vi "groups_names_query_maker.vi"(2 "Small?":bool, 3 "Name Array":string[](array[string]), 4 "Group  Name":string) -> (0 "Parameters":string[](array[string]), 1 "Group and Names Query":string)   [LabVIEW 2013]
doc: "IMPORTANT: All input values can be left unwired, and the query will be modified to suit.\nTakes the experiment group and experiment names of a query and puts them in SQL syntax, in the following pattern:\n\"\n AND\n groups.group_names = '/Group Name/'\n AND\n (experiment_settings.tag = '/Name 1/'\n OR\n experiment_settings.tag = '/Name 2/')\""
uses:
  <userlib>/_OpenG.lib/string/string.llb/Trim Whitespace (String Array)__ogtk.vi
  <userlib>/_OpenG.lib/array/array.llb/Search 1D Array (String)__ogtk.vi
  <userlib>/_OpenG.lib/array/array.llb/Delete Elements from 1D Array (String)__ogtk.vi
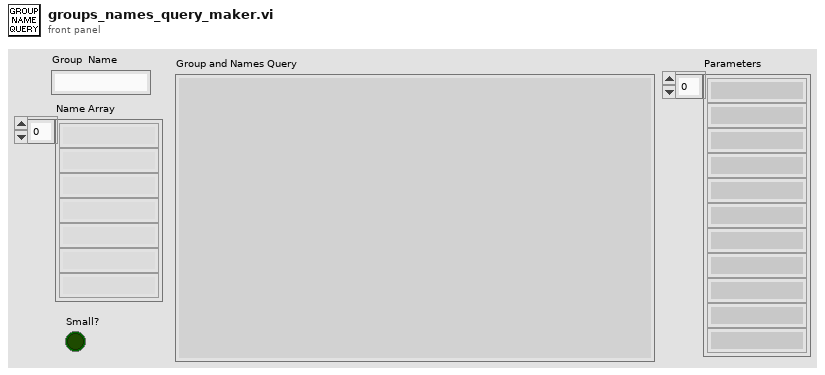
[diagram p1: front panel]
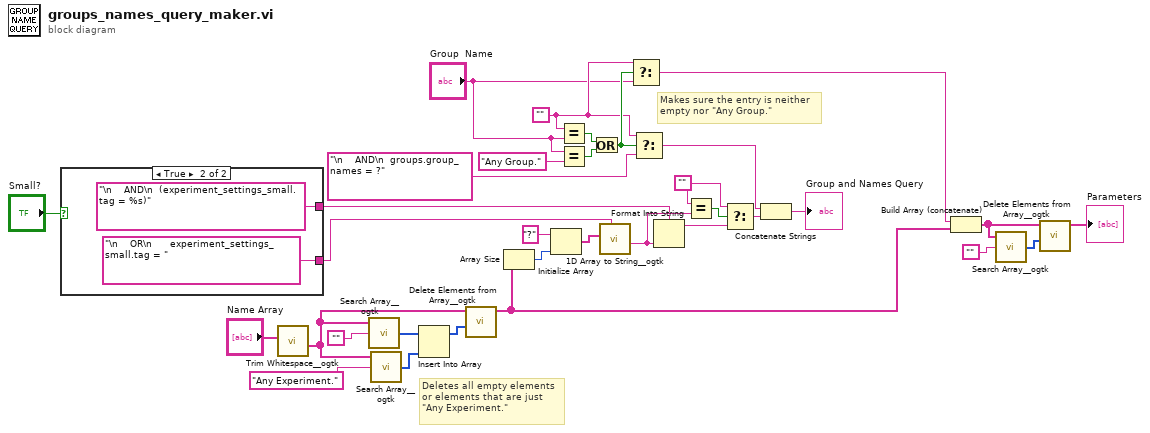
[diagram p0: block diagram]
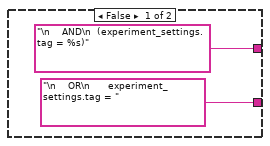
[diagram p2: hidden frame]
diagram:
  w12 = "" ("t")
  w29 = "" ("t")
  # "Makes sure the entry is neither\nempty nor \"Any Group.\""
  # "Deletes all empty elements\nor elements that are just\n\"Any Experiment.\""
  n1 = case shown="True" "Small?" {
    tunnel: ["\n    AND\n  (experiment_settings.tag = %s)" ("string") "\n    AND\n  (experiment_settings_small.tag = %s)" ("string")] -> w23
    tunnel: ["\n    OR\n      experiment_settings.tag = " ("string") "\n    OR\n      experiment_settings_small.tag = " ("string")] -> w22
    frame False {
    }
    frame True {
    }
  }
  n2 = call-poly <userlib>:"Trim Whitespace__ogtk.vi"("String in"="Name Array") -> ("String out"=w5:string[])  [unwired: 6 in]
  n3 = call-poly <userlib>:"Search Array__ogtk.vi"("Array"=w5, "Element Data"="") -> ("Indices of Elements"=w31:i32[])  [unwired: 7 in]
  n4 = call-poly <userlib>:"Search Array__ogtk.vi"("Array"=w5, "Element Data"="Any Experiment.") -> ("Indices of Elements"=w32:i32[])  [unwired: 7 in]
  n5 = Insert Into Array(array=w31, new element=w32) -> (w33:i32[])  [unwired: 1 in]
  n6 = call-poly <userlib>:"Delete Elements from Array__ogtk.vi"("indices"=w33, "array"=w5) -> ("array w/ subset deleted"=w8:string[])  [unwired: 8 in, 1 out]
  n7 = Array Size(array=w8) -> (size(s)=w9:i32)
  n8 = Initialize Array("?" ("Element Data"), w9) -> (w6:string[])
  n9 = Equal?(x=w12, y="Group  Name") -> (x = y?=w15:bool)
  n10 = Equal?(x="Group  Name", y="Any Group.") -> (x = y?=w16:bool)
  n11 = Or(x=w15, y=w16) -> (x .or. y?=w13:bool)
  n12 = call <userlib>:"1D Array to String__ogtk.vi"("delimiter (Tab)"=w22, "Array of Strings"=w6) -> ("delimited string"=w30:string)  [unwired: 9 in]
  n13 = Select(t=w12, s=w13, f="Group  Name") -> (s? t:f=w10:string)
  n14 = Select(t=w12, s=w13, f="\n    AND\n  groups.group_names = ?" ("string")) -> (s? t:f=w19:string)
  n15 = Format Into String(format string=w23, w30) -> (resulting string=w26:string)  [unwired: 2 in, 1 out]
  n16 = Equal?(x=w29, y=w30) -> (x = y?=w25:bool)
  n17 = Select(t=w29, s=w25, f=w26) -> (s? t:f=w20:string)
  n18 = Concatenate Strings(w19, w20) -> (→"Group and Names Query":string)
  n19 = Build Array (concatenate)(w10, w8) -> (w2:string[])
  n20 = call-poly <userlib>:"Search Array__ogtk.vi"("Array"=w2, "Element Data"="") -> ("Indices of Elements"=w3:i32[])  [unwired: 7 in]
  n21 = call-poly <userlib>:"Delete Elements from Array__ogtk.vi"("indices"=w3, "array"=w2) -> ("array w/ subset deleted"=→"Parameters":string[])  [unwired: 8 in, 1 out]
